vi "constructCommand_UE.vi"(6 "Time Stamp":timestamp, 8 "error in (no error)":errorcluster, 9 "svValue":variant, 11 "DataListenerThisComponent in":refnum<class "DataListenerThisComponent.lvclass">) -> (0 "error out":errorcluster, 1 "validIsTrue":bool, 2 "command":refnum<class "Command.lvclass">, 3 "DataListenerThisComponent out":refnum<class "DataListenerThisComponent.lvclass">)   [LabVIEW 2015]
doc: "Turns received shared variable information (from SubDataSVs) into commands (for the Command SV)."
uses:
  ComponentTemplateCore/ComponentModel/ComponentModel/DataListener/DataListener.lvclass
  Typedefs/CommandValue.ctl
  Typedefs/EXATypedefs.lvlib
  ICommandFactory/ICommandFactory.lvclass
  UserEventsThisComponent/UserEventsThisComponent.lvclass
  ComponentTemplateCore/ComponentModel/ComponentModel/Command/Command.lvclass
  DataListenerThisComponent.lvclass
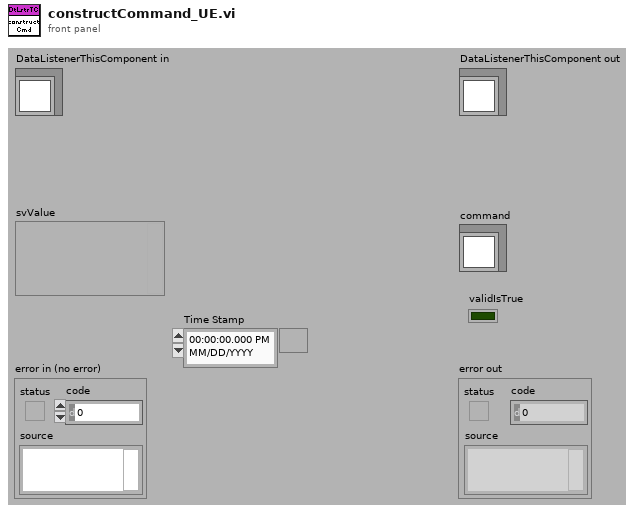
[diagram p1: front panel]
types:
  T1 = typedef "EXATypedefs.lvlib/SubDataEvents.ctl" = cluster{"ClearError":refnum<user-event>, "Disable":refnum<user-event>, "Enable":refnum<user-event>, "Exit":refnum<user-event>, "GoToStandby":refnum<user-event>, "HeartbeatIn":refnum<user-event>, "Start":refnum<user-event>}
  T2 = typedef "EXATypedefs.lvlib/CommandValue.ctl" = enum16{"ClearError", "Disable", "Enable", "Exit", "GoToStandby", "OnHeartbeat", "OnIncomingMessagingError", "OnInterrupt", "Start"}
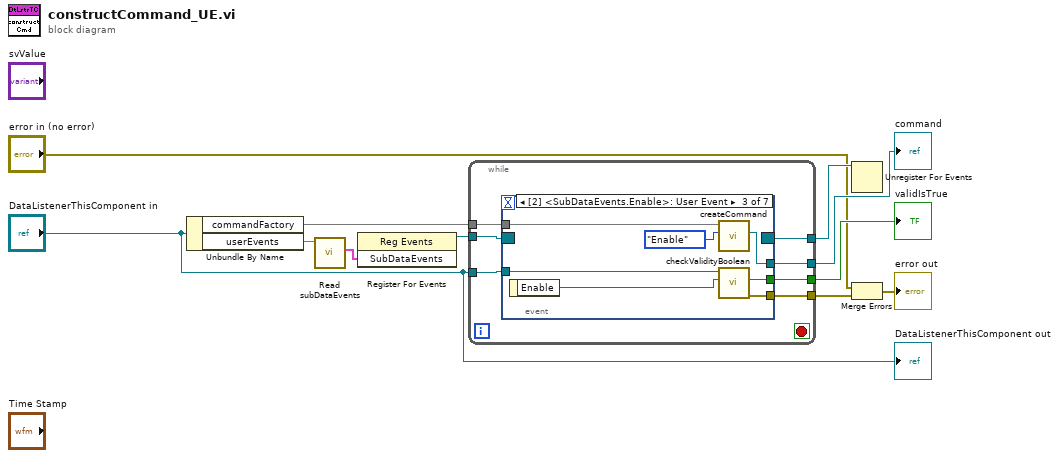
[diagram p0: block diagram]
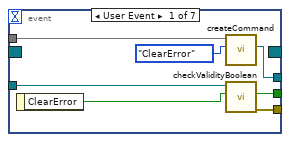
[diagram p2: hidden frame]
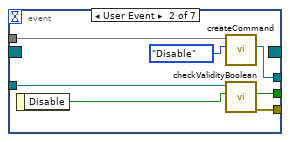
[diagram p3: hidden frame]
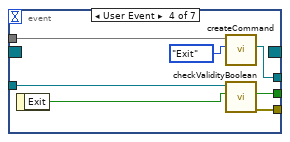
[diagram p4: hidden frame]
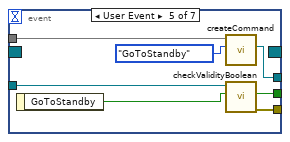
[diagram p5: hidden frame]
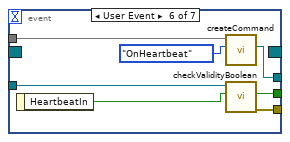
[diagram p6: hidden frame]
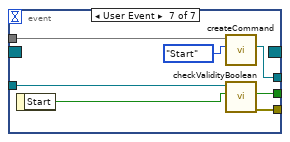
[diagram p7: hidden frame]
diagram:
  n1 = Unbundle By Name("DataListenerThisComponent in") -> ("commandFactory"=w1, "userEvents"=w10)
  n2 = call "Read subDataEvents.vi"("UserEventsThisComponent in"=w10) -> ("SubDataEvents"=w8:T1)  [unwired: 9 in, 1 out]
  n3 = register-events(w8) -> (reference out=w9:refnum<event-registration>)  [unwired: 2 in, 1 out]
  n4 = while {
    tunnel: w9 -> [w18]
    tunnel: "DataListenerThisComponent in" -> [w17]
    tunnel: [w16] -> w6
    tunnel: [w15] -> w5
    tunnel: [w14] -> w4
    tunnel: [w13] -> w2
    tunnel: w1 -> [w12]
    stop <- _ stop-if-true
    n5 = event shown="[2] <SubDataEvents.Enable>: User Event" {
      selector: w18 -> [_ _ _ _ _ _ _]
      dyn-events: [_ _ _ _ _ _ _] -> w14
      timeout: _ -> [_ _ _ _ _ _ _]
      tunnel: w17 -> [w23 w30 w37 w44 w51 w58 w65]
      tunnel: [w22 w29 w36 w43 w50 w57 w64] -> w16
      tunnel: [w21 w28 w35 w42 w49 w56 w63] -> w13
      tunnel: [w20 w27 w34 w41 w48 w55 w62] -> w15
      tunnel: w12 -> [w19 w26 w33 w40 w47 w54 w61]
      event User Event {
        n6 = event-data() -> ("ClearError"=w24:bool)  [unwired: 1 in]
        n7 = call-dynamic "createCommand.vi"("commandValue"=CommandValue."ClearError", "ICommandFactory in"=w19) -> ("command"=w20:refnum<class "Command.lvclass">)  [unwired: 7 in, 2 out]
        n8 = call "checkValidityBoolean.vi"("svValue"=w24, "DataListener in"=w23) -> ("error out"=w21:errorcluster, "validIsTrue"=w22:bool)  [unwired: 7 in, 1 out]
      }
      event User Event {
        n9 = event-data() -> ("Disable"=w31:bool)  [unwired: 1 in]
        n10 = call-dynamic "createCommand.vi"("commandValue"=CommandValue."Disable", "ICommandFactory in"=w26) -> ("command"=w27:refnum<class "Command.lvclass">)  [unwired: 7 in, 2 out]
        n11 = call "checkValidityBoolean.vi"("svValue"=w31, "DataListener in"=w30) -> ("error out"=w28:errorcluster, "validIsTrue"=w29:bool)  [unwired: 7 in, 1 out]
      }
      event User Event {
        n12 = event-data() -> ("Enable"=w38:bool)  [unwired: 1 in]
        n13 = call-dynamic "createCommand.vi"("commandValue"=CommandValue."Enable", "ICommandFactory in"=w33) -> ("command"=w34:refnum<class "Command.lvclass">)  [unwired: 7 in, 2 out]
        n14 = call "checkValidityBoolean.vi"("svValue"=w38, "DataListener in"=w37) -> ("error out"=w35:errorcluster, "validIsTrue"=w36:bool)  [unwired: 7 in, 1 out]
      }
      event User Event {
        n15 = event-data() -> ("Exit"=w45:bool)  [unwired: 1 in]
        n16 = call-dynamic "createCommand.vi"("commandValue"=CommandValue."Exit", "ICommandFactory in"=w40) -> ("command"=w41:refnum<class "Command.lvclass">)  [unwired: 7 in, 2 out]
        n17 = call "checkValidityBoolean.vi"("svValue"=w45, "DataListener in"=w44) -> ("error out"=w42:errorcluster, "validIsTrue"=w43:bool)  [unwired: 7 in, 1 out]
      }
      event User Event {
        n18 = event-data() -> ("GoToStandby"=w52:bool)  [unwired: 1 in]
        n19 = call-dynamic "createCommand.vi"("commandValue"=CommandValue."GoToStandby", "ICommandFactory in"=w47) -> ("command"=w48:refnum<class "Command.lvclass">)  [unwired: 7 in, 2 out]
        n20 = call "checkValidityBoolean.vi"("svValue"=w52, "DataListener in"=w51) -> ("error out"=w49:errorcluster, "validIsTrue"=w50:bool)  [unwired: 7 in, 1 out]
      }
      event User Event {
        n21 = event-data() -> ("HeartbeatIn"=w59:bool)  [unwired: 1 in]
        n22 = call-dynamic "createCommand.vi"("commandValue"=CommandValue."OnHeartbeat", "ICommandFactory in"=w54) -> ("command"=w55:refnum<class "Command.lvclass">)  [unwired: 7 in, 2 out]
        n23 = call "checkValidityBoolean.vi"("svValue"=w59, "DataListener in"=w58) -> ("error out"=w56:errorcluster, "validIsTrue"=w57:bool)  [unwired: 7 in, 1 out]
      }
      event User Event {
        n24 = event-data() -> ("Start"=w66:bool)  [unwired: 1 in]
        n25 = call-dynamic "createCommand.vi"("commandValue"=CommandValue."Start", "ICommandFactory in"=w61) -> ("command"=w62:refnum<class "Command.lvclass">)  [unwired: 7 in, 2 out]
        n26 = call "checkValidityBoolean.vi"("svValue"=w66, "DataListener in"=w65) -> ("error out"=w63:errorcluster, "validIsTrue"=w64:bool)  [unwired: 7 in, 1 out]
      }
    }
  }
  "command" <- w5
  "validIsTrue" <- w6
  n27 = Unregister For Events(event registration refnum=w4) -> ()  [unwired: 1 in, 1 out]
  n28 = Merge Errors("error in (no error)", w2) -> (→"error out":errorcluster)
  "DataListenerThisComponent out" <- "DataListenerThisComponent in"
